vi "Perform_large_file_Analysis.vi"(0 "IntensityGraph in":refnum<vi>) -> (1 "size(s)":i32, 2 "Analysis_Data":T2, 3 "Spectrum Data":T1, 4 "Discr. Slope":cluster{"Array":dbl[], "Array":dbl[]})   [LabVIEW 2015]
uses:
  ESA_Data_Analysis_Global_VIs.vi
  <vilib>/Analysis/NI_AALPro.lvlib
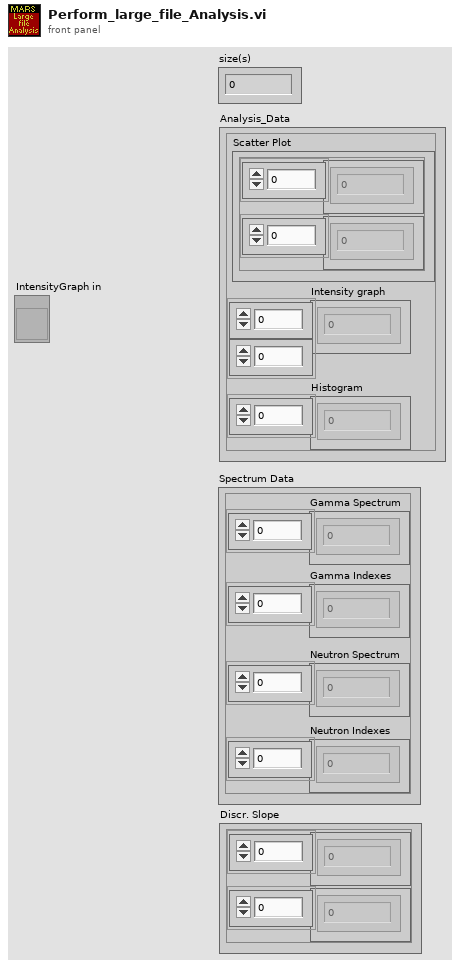
[diagram p1: front panel]
types:
  T1 = cluster{"Gamma Spectrum":dbl[], "Gamma Indexes":i32[], "Neutron Spectrum":dbl[], "Neutron Indexes":i32[]}
  T2 = cluster{"Scatter Plot":cluster{"Array":dbl[], "Array":dbl[]}, "Intensity graph":u32[][], "Histogram":u32[]}
  T3 = cluster{"Cursor.Cursor X1":dbl, "Cursor.Cursor Y1":dbl, "Cursor.Cursor X2":dbl, "Cursor.Cursor Y2":dbl}
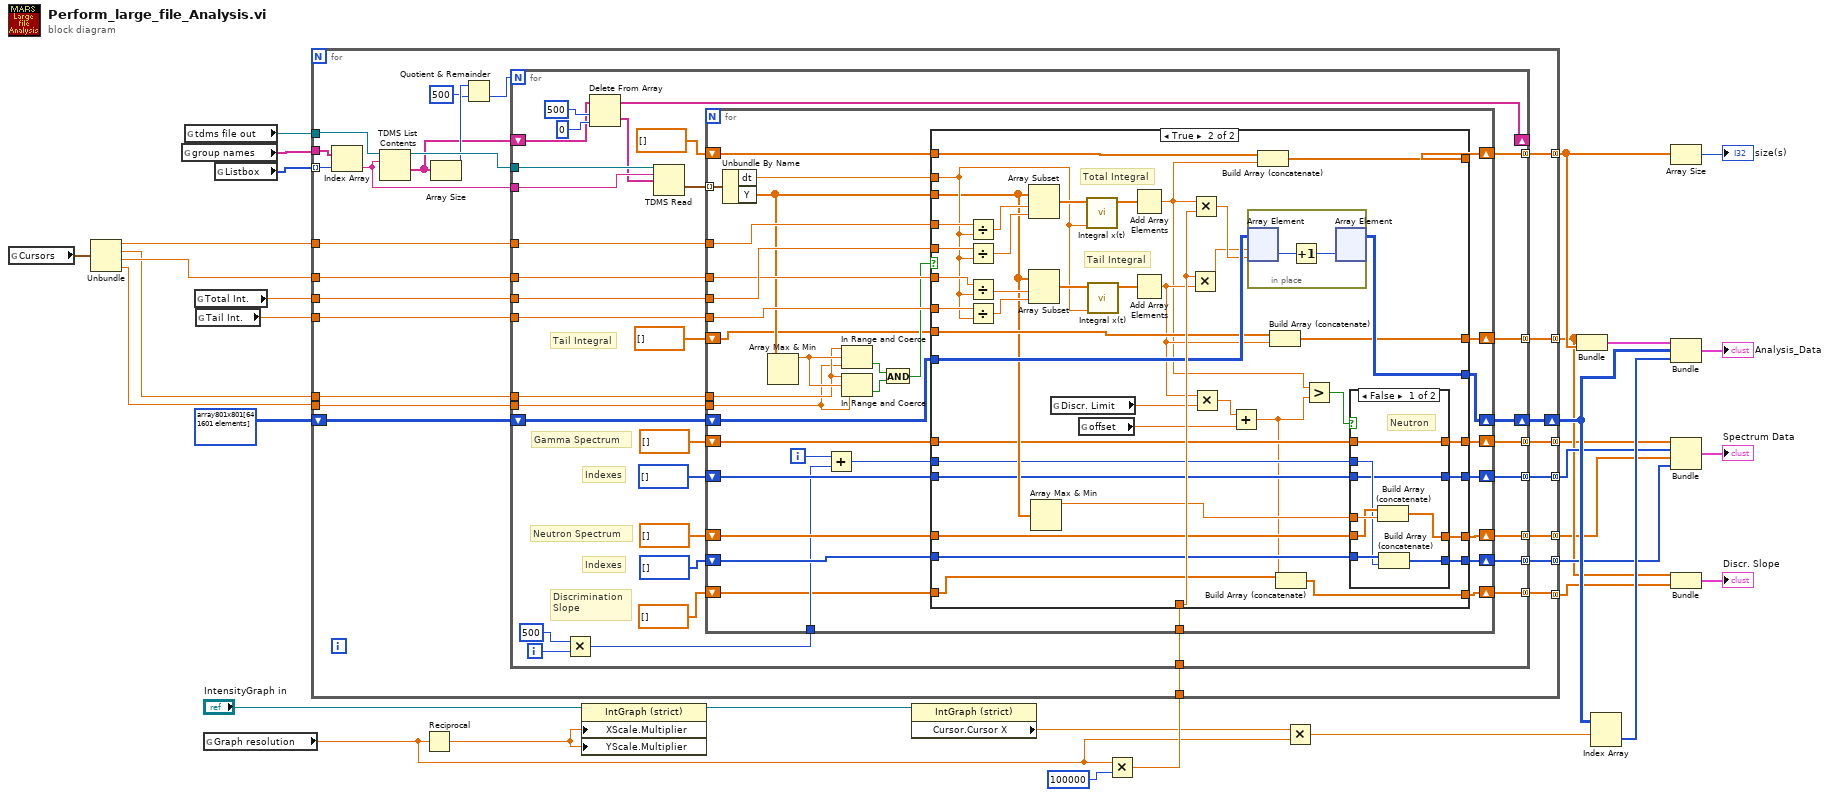
[diagram p0: block diagram]
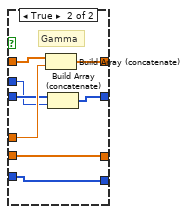
[diagram p3: hidden frame]
diagram:
  n1 = global read "ESA_Data_Analysis_Global_VIs.vi" "Cursors"() -> (w10:T3)
  n2 = Unbundle(w10) -> ("Cursor.Cursor X1"=w23:dbl, "Cursor.Cursor Y1"=w21:dbl, "Cursor.Cursor X2"=w22:dbl, "Cursor.Cursor Y2"=w20:dbl)
  n3 = global read "ESA_Data_Analysis_Global_VIs.vi" "group names"() -> (w12:string[])
  n4 = global read "ESA_Data_Analysis_Global_VIs.vi" "tdms file out"() -> (w13:refnum<k34>)
  n5 = global read "ESA_Data_Analysis_Global_VIs.vi" "Total Int."() -> (w16:dbl)
  n6 = global read "ESA_Data_Analysis_Global_VIs.vi" "Tail Int."() -> (w15:dbl)
  n7 = global read "ESA_Data_Analysis_Global_VIs.vi" "Graph resolution"() -> (w14:dbl)
  n8 = global read "ESA_Data_Analysis_Global_VIs.vi" "Listbox"() -> (w11:i32[])
  n9 = Reciprocal(x=w14) -> (1/x=w32:dbl)
  n10 = property on="Property Node" class="IntGraph (strict)"(reference="IntensityGraph in", "XScale.Multiplier"=w32, "YScale.Multiplier"=w32) -> (reference out=w28:refnum<vi>)  [unwired: 1 in, 1 out]
  n11 = property on="Property Node" class="IntGraph (strict)"(reference=w28) -> ("Cursor.Cursor X"=w27:dbl)  [unwired: 1 in, 2 out]
  n12 = Multiply(x=w14, y=100000) -> (x*y=w30:dbl)
  n13 = for {
    tunnel: w13 -> [w58]
    tunnel: w12 -> [w56]
    tunnel: w11 -> [w55] mode=indexing
    tunnel: w23 -> [w51]
    tunnel: w22 -> [w50]
    tunnel: w16 -> [w49]
    tunnel: w15 -> [w48]
    tunnel: w30 -> [w47]
    shift-right: [w45] -> w19
    shift-left: u32[][] array801x801[641601 elements] -> [w46]
    tunnel: [w44] -> w25 mode=concatenating
    tunnel: [w43] -> w4 mode=concatenating
    tunnel: w21 -> [w40]
    tunnel: w20 -> [w39]
    tunnel: [w38] -> w1 mode=concatenating
    tunnel: [w37] -> w2 mode=concatenating
    tunnel: [w36] -> w9 mode=concatenating
    tunnel: [w35] -> w8 mode=concatenating
    tunnel: [w34] -> w5 mode=concatenating
    n14 = Index Array(array=w56, index=w55) -> (element=w52:string)
    n15 = TDMS List Contents(6:w52, 7:w58) -> (1:w42:string[], 3:w57:refnum<k34>)  [unwired: 1 in, 2 out]
    n16 = Array Size(array=w42) -> (size(s)=w54:i32)
    n17 = Quotient & Remainder(x=w54, y=500) -> (floor(x/y)=w41:i32)  [unwired: 1 out]
    n18 = for {
      N: w41 -> [_]
      tunnel: w57 -> [w92]
      tunnel: w52 -> [w81]
      tunnel: w51 -> [w90]
      tunnel: w50 -> [w89]
      tunnel: w49 -> [w88]
      tunnel: w48 -> [w87]
      tunnel: w47 -> [w86]
      shift-right: [w84] -> w45
      shift-left: w46 -> [w85]
      tunnel: [w83] -> w44 mode=concatenating
      tunnel: [w82] -> w43 mode=concatenating
      shift-right: [w77] -> _
      shift-left: w42 -> [w78]
      tunnel: w40 -> [w75]
      tunnel: w39 -> [w74]
      tunnel: [w69] -> w38 mode=concatenating
      tunnel: [w68] -> w37 mode=concatenating
      tunnel: [w66] -> w36 mode=concatenating
      tunnel: [w64] -> w35 mode=concatenating
      tunnel: [w59] -> w34 mode=concatenating
      i -> [w63]
      # "Tail Integral"
      # "Discrimination\nSlope"
      # "Indexes"
      # "Indexes"
      # "Neutron Spectrum"
      # "Gamma Spectrum"
      n19 = Multiply(x=500, y=w63) -> (x*y=w62:i32)
      n20 = Delete From Array(array=w78, length=500, index=0) -> (deleted portion=w76:string[], array with subset deleted=w77:string[])
      n21 = TDMS Read(0:w92, 5:w81, 7:w76) -> (10:w91:waveform(dbl)[])  [unwired: 5 in, 5 out]
      n22 = for {
        tunnel: w91 -> [w125] mode=indexing
        tunnel: w90 -> [w124]
        tunnel: w88 -> [w123]
        tunnel: w89 -> [w122]
        tunnel: w87 -> [w121]
        tunnel: w86 -> [w119]
        shift-right: [w117] -> w84
        shift-left: w85 -> [w118]
        tunnel: w75 -> [w109]
        tunnel: w74 -> [w108]
        shift-right: [w116] -> w83
        shift-left: dbl[] [] -> [w107]
        shift-right: [w115] -> w82
        shift-left: dbl[] [] -> [w106]
        shift-right: [w104] -> w69
        shift-left: dbl[] [] -> [w105]
        shift-right: [w102] -> w68
        shift-left: dbl[] [] -> [w103]
        shift-right: [w99] -> w66
        shift-left: i32[] [] -> [w101]
        shift-right: [w97] -> w64
        shift-left: i32[] [] -> [w98]
        tunnel: w62 -> [w95]
        shift-right: [w93] -> w59
        shift-left: dbl[] [] -> [w94]
        i -> [w100]
        n23 = Unbundle By Name(w125) -> ("dt"=w120:dbl, "Y"=w114:dbl[])
        n24 = Array Max & Min(array=w114) -> (max value=w113:dbl)  [unwired: 3 out]
        n25 = Add(x=w100, y=w95) -> (x+y=w96:i32)
        n26 = In Range and Coerce(upper limit=w109, x=w113, lower limit=w108) -> (In Range?=w112:bool)  [unwired: 1 out]
        n27 = In Range and Coerce(upper limit=w109, x=w113, lower limit=w108) -> (In Range?=w111:bool)  [unwired: 1 out]
        n28 = And(x=w112, y=w111) -> (x .and. y?=w110:bool)
        n29 = case shown="True" w110 {
          tunnel: w124 -> [_ w171]
          tunnel: w123 -> [_ w170]
          tunnel: w122 -> [_ w169]
          tunnel: w121 -> [_ w168]
          tunnel: w114 -> [_ w155]
          tunnel: w120 -> [_ w163]
          tunnel: w119 -> [_ w162]
          tunnel: w118 -> [w131 w161]
          tunnel: [w131 w160] -> w117
          tunnel: [w133 w159] -> w116
          tunnel: [w132 w157] -> w115
          tunnel: w107 -> [w133 w158]
          tunnel: w106 -> [w132 w156]
          tunnel: w105 -> [w130 w151]
          tunnel: [w130 w150] -> w104
          tunnel: w103 -> [w129 w149]
          tunnel: [w129 w148] -> w102
          tunnel: w101 -> [w128 w146]
          tunnel: w96 -> [_ w145]
          tunnel: [w128 w144] -> w99
          tunnel: w98 -> [w127 w143]
          tunnel: [w127 w142] -> w97
          tunnel: w94 -> [w126 w138]
          tunnel: [w126 w137] -> w93
          frame False {
          }
          frame True {
            # "Total Integral"
            # "Tail Integral"
            n30 = Divide(x=w171, y=w163) -> (x/y=w175:dbl)
            n31 = Divide(x=w170, y=w163) -> (x/y=w174:dbl)
            n32 = Divide(x=w169, y=w163) -> (x/y=w172:dbl)
            n33 = Divide(x=w168, y=w163) -> (x/y=w173:dbl)
            n34 = Array Subset(array=w155, index=w175, length=w174) -> (w164:dbl[])
            n35 = Array Subset(array=w155, index=w172, length=w173) -> (w167:dbl[])
            n36 = Array Max & Min(array=w155) -> (max value=w152:dbl)  [unwired: 3 out]
            n37 = global read "ESA_Data_Analysis_Global_VIs.vi" "Discr. Limit"() -> (w147:dbl)
            n38 = global read "ESA_Data_Analysis_Global_VIs.vi" "offset"() -> (w139:dbl)
            n39 = call <vilib>:"Integral x(t).vi"("dt"=w163, "X"=w164) -> ("Integral X"=w166:dbl[])  [unwired: 8 in, 1 out]
            n40 = call <vilib>:"Integral x(t).vi"("dt"=w163, "X"=w167) -> ("Integral X"=w165:dbl[])  [unwired: 8 in, 1 out]
            n41 = Add Array Elements(numeric array=w166) -> (sum=w134:dbl)
            n42 = Add Array Elements(numeric array=w165) -> (sum=w135:dbl)
            n43 = Multiply(x=w162, y=w135) -> (x*y=w141:dbl)
            n44 = Multiply(x=w134, y=w162) -> (x*y=w154:dbl)
            n45 = Multiply(x=w135, y=w147) -> (x*y=w140:dbl)
            n46 = Add(x=w140, y=w139) -> (x+y=w136:dbl)
            n47 = in-place {
              n48 = in-place-array #1(w161, w141, w154) -> (w193:u32)
              n49 = Increment(x=w193) -> (x+1=w192:u32)
              n50 = in-place-array #1(w192) -> (w160:u32[][])  [unwired: 2 out]
            }
            n51 = Build Array (concatenate)(w158, w134) -> (w159:dbl[])
            n52 = Build Array (concatenate)(w156, w135) -> (w157:dbl[])
            n53 = Build Array (concatenate)(w138, w136) -> (w137:dbl[])
            n54 = Greater?(x=w134, y=w136) -> (0:w153:bool)
            n55 = case shown="False" w153 {
              tunnel: w152 -> [w183 w191]
              tunnel: [w181 w190] -> w150
              tunnel: w151 -> [w181 w189]
              tunnel: w149 -> [w182 w188]
              tunnel: [w180 w188] -> w148
              tunnel: w146 -> [w176 w187]
              tunnel: w145 -> [w178 w186]
              tunnel: [w176 w185] -> w144
              tunnel: w143 -> [w179 w184]
              tunnel: [w177 w184] -> w142
              frame False {
                # "Neutron"
                n56 = Build Array (concatenate)(w182, w183) -> (w180:dbl[])
                n57 = Build Array (concatenate)(w179, w178) -> (w177:i32[])
              }
              frame True {
                # "Gamma"
                n58 = Build Array (concatenate)(w189, w191) -> (w190:dbl[])
                n59 = Build Array (concatenate)(w187, w186) -> (w185:i32[])
              }
            }
          }
        }
      }
    }
  }
  n60 = Multiply(x=w27, y=w14) -> (x*y=w33:dbl)
  n61 = Bundle(w4, w25) -> (w6:cluster{dbl[], dbl[]})  [unwired: 1 in]
  n62 = Index Array(array=w19, index (row)=w33) -> (element=w18:u32[])  [unwired: 1 in]
  n63 = Array Size(array=w25) -> (size(s)=→"size(s)":i32)
  n64 = Bundle(w6, w19, w18) -> (→"Analysis_Data":cluster{cluster{dbl[], dbl[]}, u32[][], u32[]})  [unwired: 1 in]
  n65 = Bundle(w1, w9, w2, w8) -> (→"Spectrum Data":cluster{dbl[], i32[], dbl[], i32[]})  [unwired: 1 in]
  n66 = Bundle(w4, w5) -> (→"Discr. Slope":cluster{dbl[], dbl[]})  [unwired: 1 in]
